vi "DrugControllerMain.vi"() -> ()   [LabVIEW 2019]
uses:
  DrugDosageTimeStampReference.ctl
panel:
  in  "TimeSimulator":dbl(slide) scale=0.0..24.0
  in  "Show Status":bool
  in  "Start":bool
  in  "Max Booster Allowed":u32 max=2
  in  "Planned Dosages":u32 max=10
  in  "Patient Name":string
  in  "Drug Id":string
  in  "Patient Id":string
  in  "Set Schedule":bool
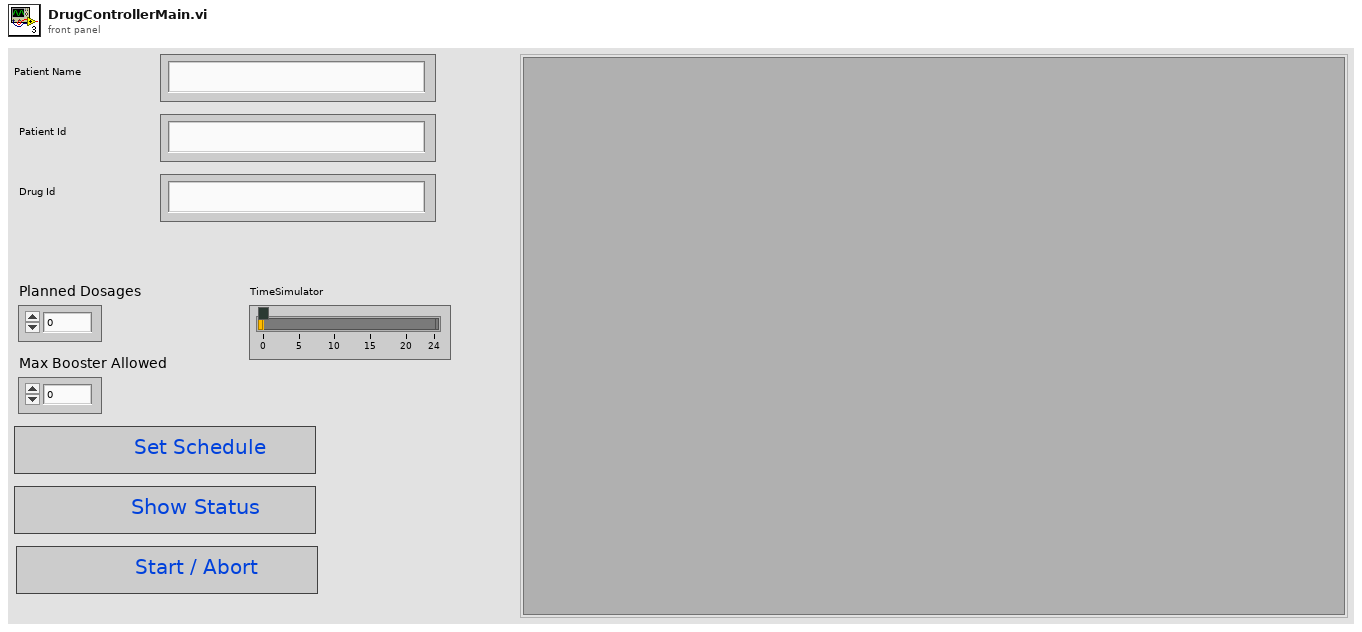
[diagram p1: front panel]
types:
  T1 = typedef "DrugDosageTimeStampReference.ctl" = cluster{"TimeStampControlReference":refnum<vi>, "DosageTime":timestamp}
  T2 = enum8{"Enabled", "Disabled", "Disabled and Grayed Out"}
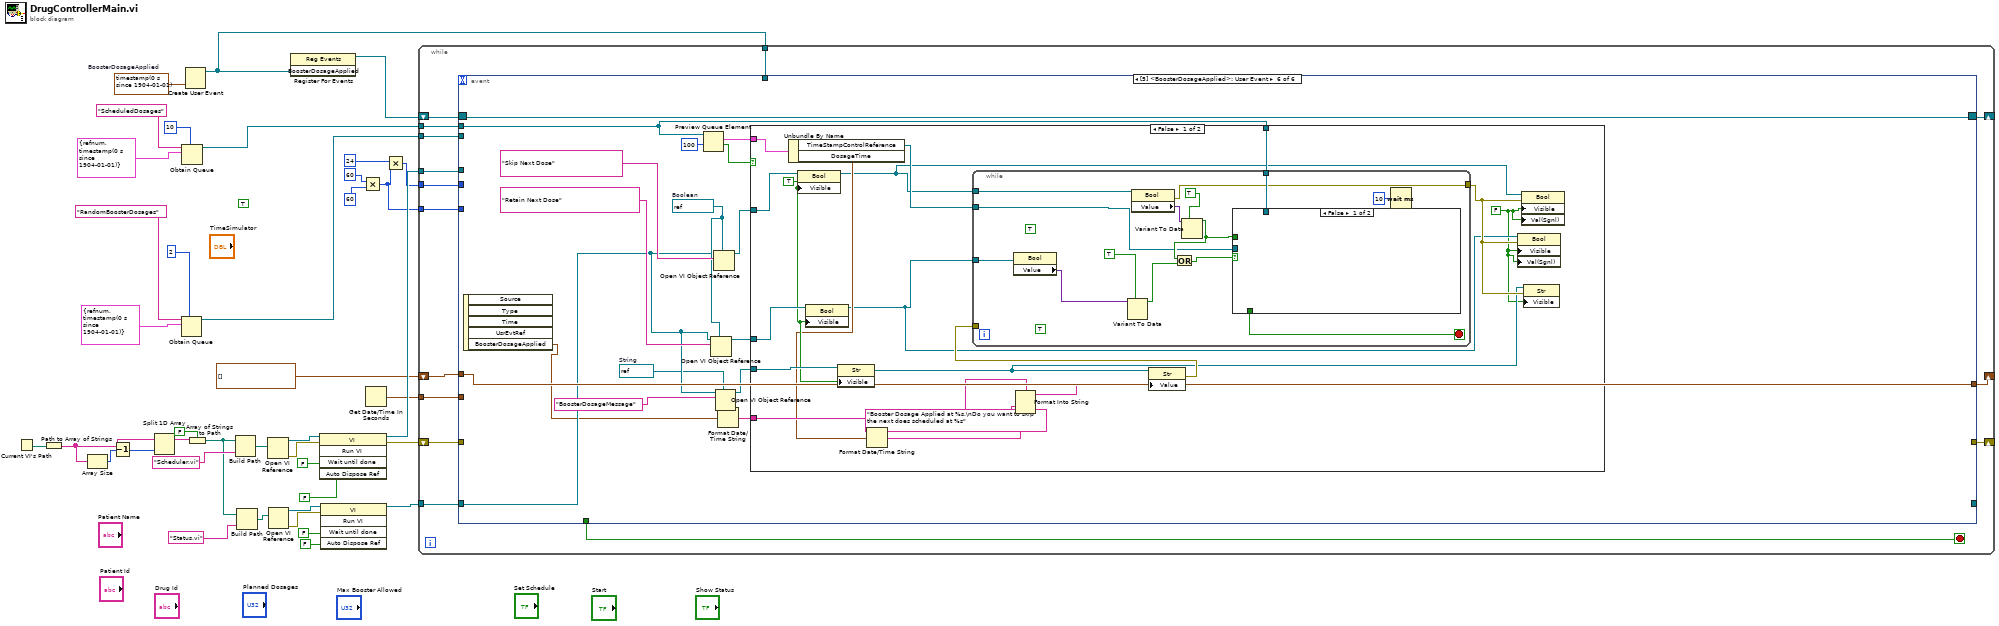
[diagram p0: block diagram]
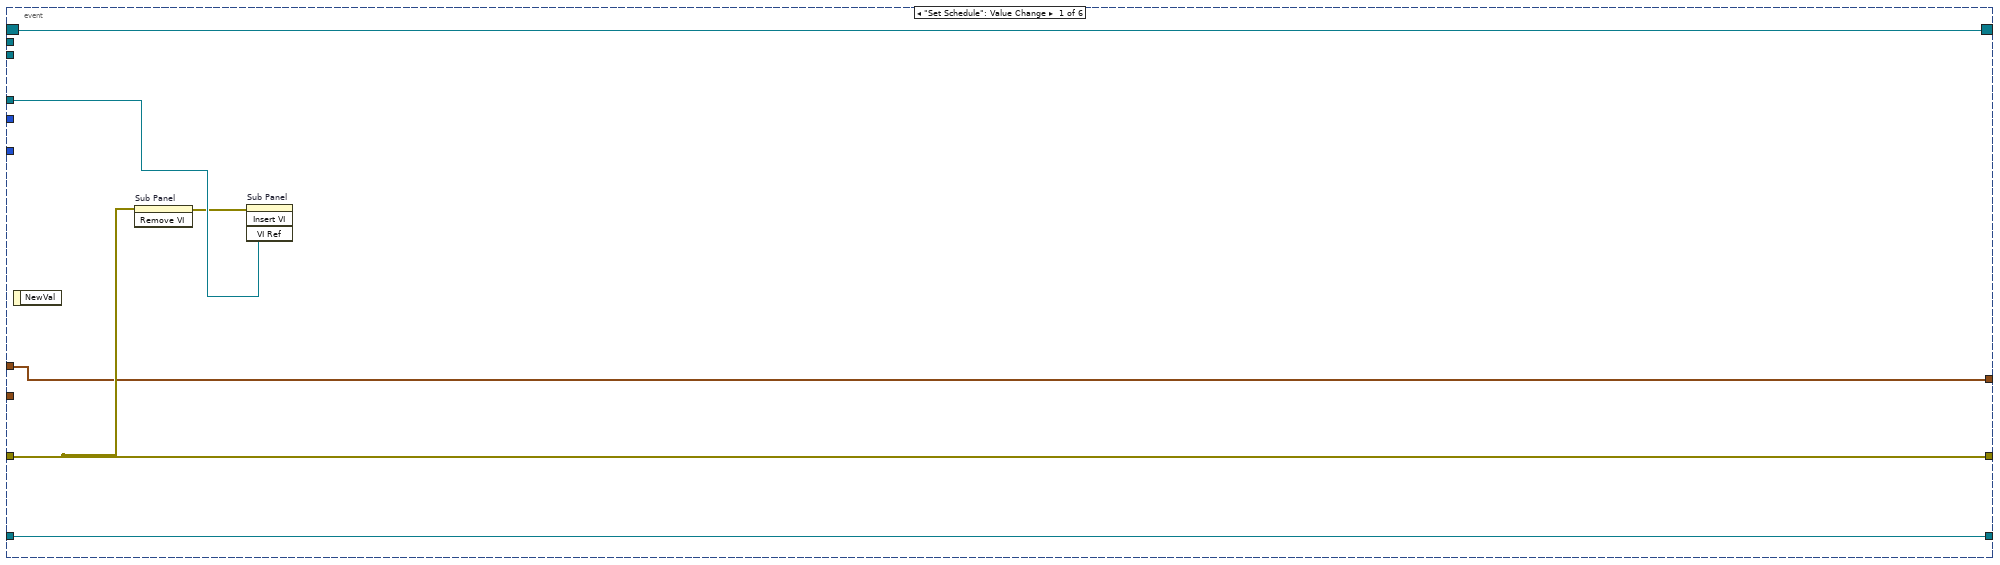
[diagram p2: hidden frame]
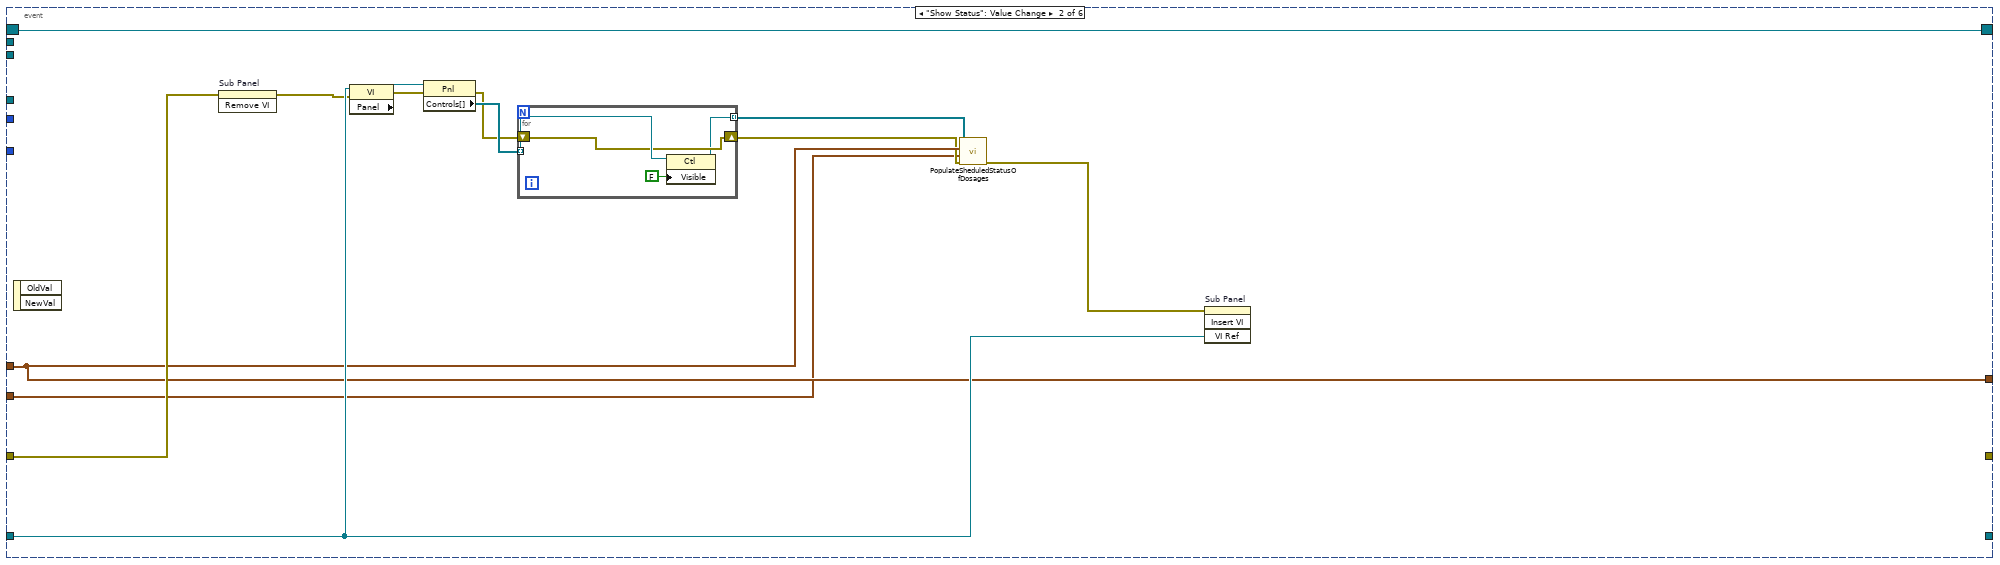
[diagram p3: hidden frame]
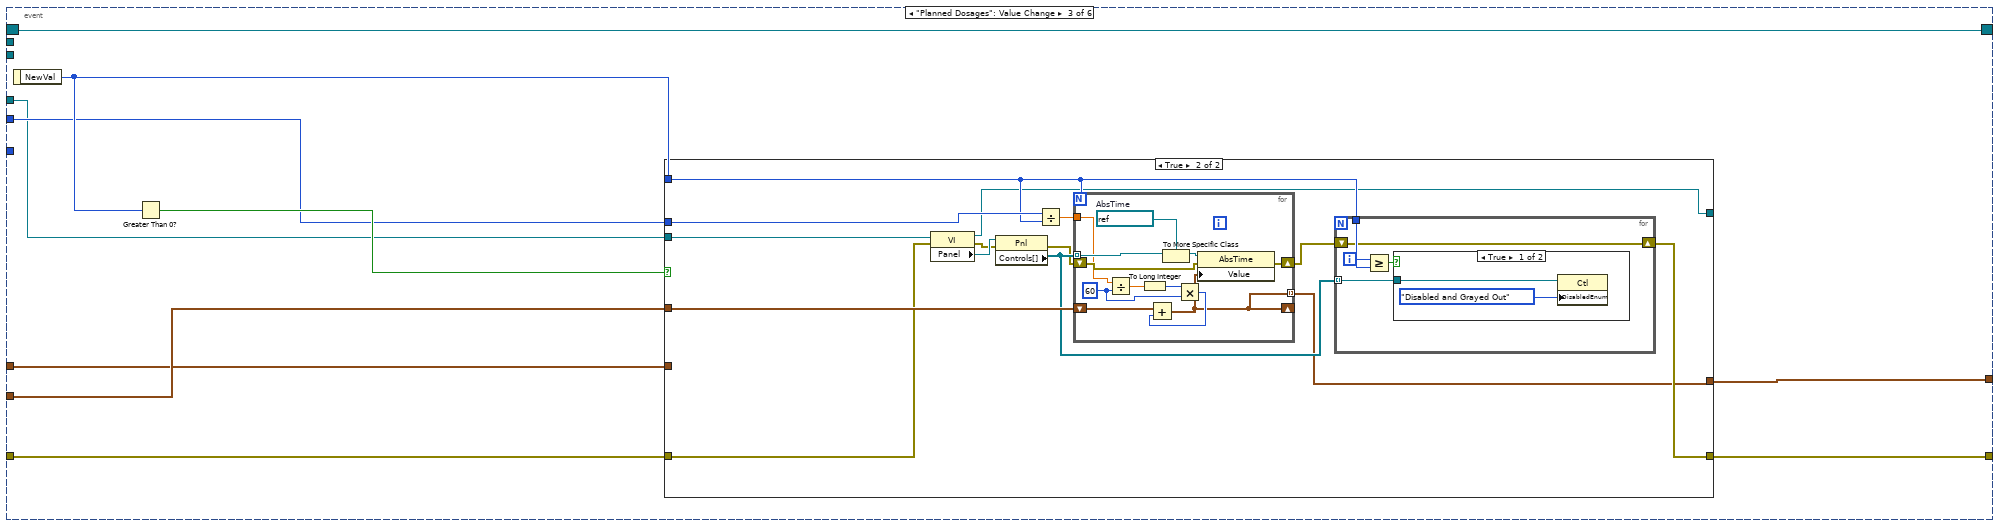
[diagram p4: hidden frame]
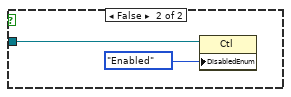
[diagram p6: hidden frame]
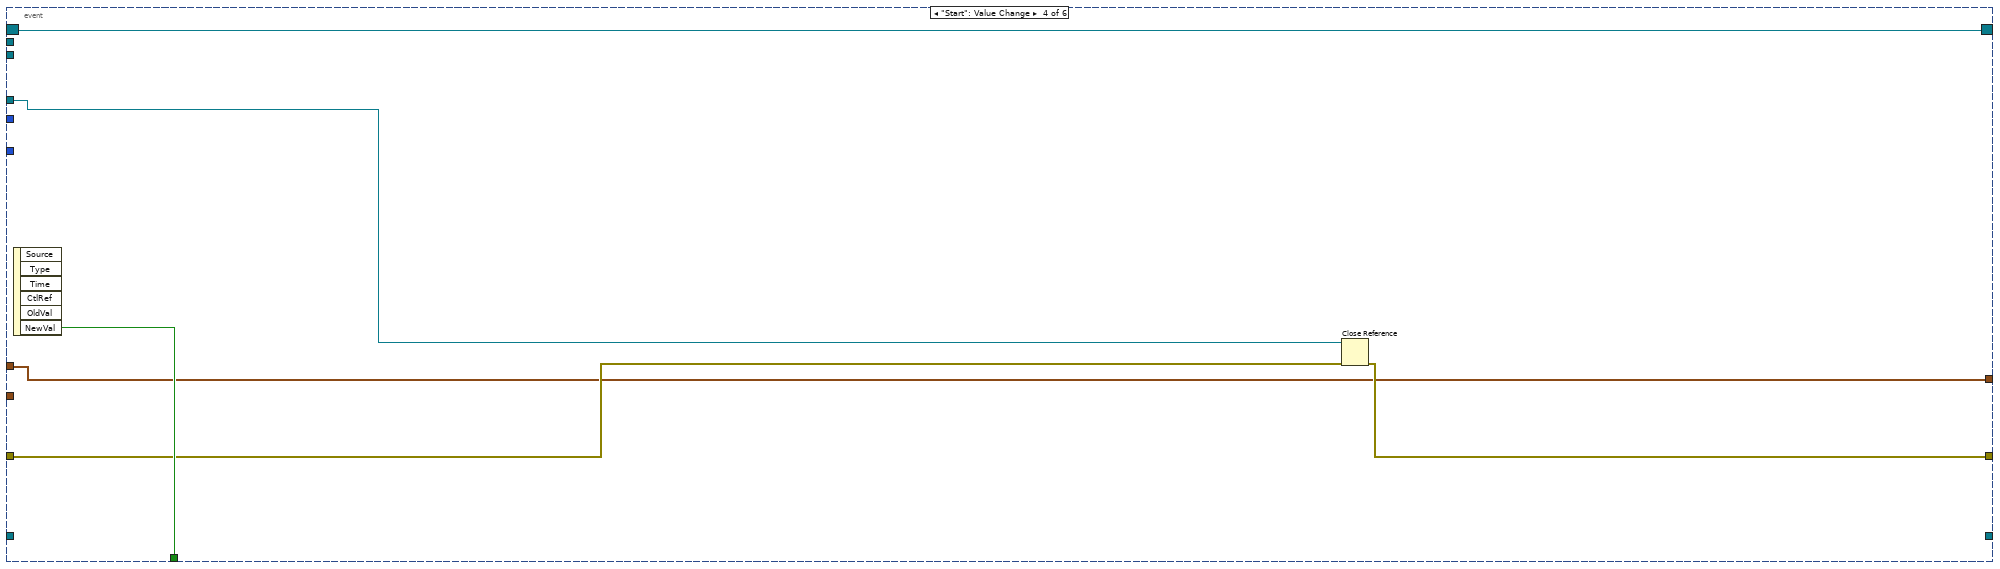
[diagram p7: hidden frame]
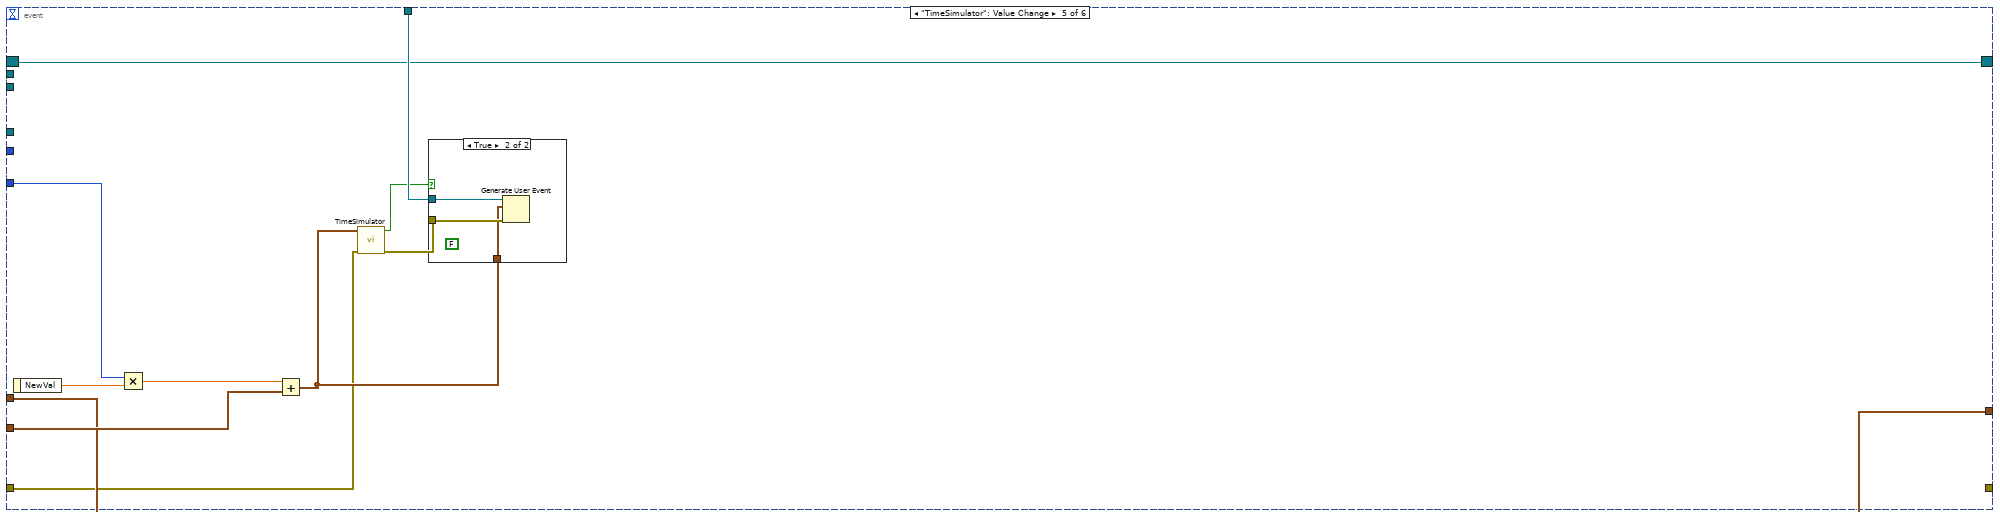
[diagram p8: hidden frame]
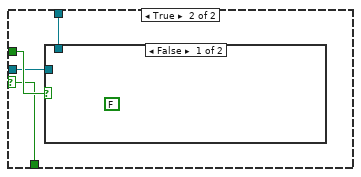
[diagram p10: hidden frame]
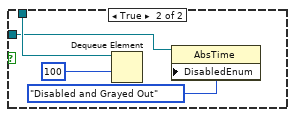
[diagram p11: hidden frame]
diagram:
  w10 = timestamp(0 s since 1904-01-01)  # BoosterDosageApplied
  (unwired) TRUE
  n1 = Current VI's Path() -> (path=w33:path)
  n2 = Path to Array of Strings(0:w33) -> (2:w35:string[])  [unwired: 1 out]
  n3 = Array Size(array=w35) -> (size(s)=w34:i32)
  n4 = Decrement(x=w34) -> (x-1=w37:i32)
  n5 = Split 1D Array(array=w35, index=w37) -> (first subarray=w38:string[])  [unwired: 1 out]
  n6 = Obtain Queue(max queue size (-1, unlimited)=2, name (unnamed)="RandomBoosterDosages", element data type=T1 {"TimeStampControlReference"=refnum, "DosageTime"=timestamp(0 s since 1904-01-01)}) -> (queue out=w1:refnum<queue>)  [unwired: 2 in, 2 out]
  n7 = Obtain Queue(max queue size (-1, unlimited)=10, name (unnamed)="ScheduledDosages", element data type=T1 {"TimeStampControlReference"=refnum, "DosageTime"=timestamp(0 s since 1904-01-01)}) -> (queue out=w6:refnum<queue>)  [unwired: 2 in, 2 out]
  n8 = Create User Event(user event datatype=w10) -> (user event=w9:refnum<user-event>)  [unwired: 1 in, 1 out]
  n9 = Array of Strings to Path(0:w38, 1:FALSE ("relative")) -> (2:w19:path)
  n10 = Build Path(base path=w19, name or relative path="Scheduler.vi") -> (appended path=w36:path)
  n11 = Build Path(base path=w19, name or relative path="Status.vi") -> (appended path=w20:path)
  n12 = Open VI Reference(vi path=w36) -> (vi reference=w27:refnum<vi>, error out=w28:errorcluster)  [unwired: 5 in]
  n13 = Open VI Reference(vi path=w20) -> (vi reference=w24:refnum<vi>, error out=w23:errorcluster)  [unwired: 5 in]
  n14 = register-events(w9) -> (reference out=w11:refnum<event-registration>)  [unwired: 2 in, 1 out]
  n15 = invoke class="VI" method="Run VI"(reference=w27, error in=w28, "Wait until done"=FALSE ("Wait Until Done"), "Auto Dispose Ref"=FALSE ("Auto Dispose Reference")) -> (reference out=w26:refnum<vi>, error out=w25:errorcluster)  [unwired: 1 in, 3 out]
  n16 = invoke class="VI" method="Run VI"(reference=w24, error in=w23, "Wait until done"=FALSE ("Wait Until Done"), "Auto Dispose Ref"=FALSE ("Auto Dispose Reference")) -> (reference out=w17:refnum<vi>)  [unwired: 1 in, 4 out]
  n17 = Multiply(x=60, y=60) -> (x*y=w14:i32)
  n18 = Get Date/Time In Seconds() -> (seconds since 1Jan1904=w12:timestamp)
  n19 = Multiply(x=24, y=w14) -> (x*y=w15:i32)
  n20 = while {
    tunnel: w15 -> [w54]
    shift-right: [w52] -> _
    shift-left: w25 -> [w51]
    tunnel: w17 -> [w50]
    tunnel: w26 -> [w53]
    tunnel: w14 -> [w49]
    tunnel: w12 -> [w48]
    shift-right: [w47] -> _
    shift-left: timestamp[] [] -> [w46]
    tunnel: w9 -> [w44]
    shift-right: [w43] -> _
    shift-left: w11 -> [w45]
    tunnel: w6 -> [w42]
    tunnel: w1 -> [w41]
    stop <- w55 stop-if-true
    n21 = event shown="[5] <BoosterDosageApplied>: User Event" {
      selector: w45 -> [w56 w62 w79 w127 w135 w162]
      dyn-events: [w56 w62 w79 w127 w135 w162] -> w43
      timeout: _ -> [_ _ _ _ _ _]
      tunnel: [_ _ _ w132 _ _] -> w55
      tunnel: w54 -> [_ _ w86 _ _ _]
      tunnel: w53 -> [w61 _ w85 w130 _ _]
      tunnel: [w60 _ w84 w131 _ _] -> w52
      tunnel: w51 -> [w60 w74 w83 w129 w133 _]
      tunnel: w50 -> [w57 w71 _ _ _ w152]
      tunnel: w49 -> [_ _ _ _ w143 _]
      tunnel: w48 -> [_ w63 w82 _ w141 _]
      tunnel: [w58 w69 w81 w128 w139 w163] -> w47
      tunnel: w46 -> [w58 w69 w80 w128 w139 w163]
      tunnel: [w57 _ _ _ _ _] -> _
      tunnel: w44 -> [_ _ _ _ w136 _]
      tunnel: w42 -> [_ _ _ _ _ w147]
      tunnel: w41 -> [_ _ _ _ _ _]
      event "Set Schedule": Value Change {
        n22 = event-data() -> ()  [unwired: 1 in, 1 out]
        n23 = invoke on="Sub Panel" class="SubPnl" method="Remove VI"(error in=w60) -> (error out=w59:errorcluster)  [unwired: 2 in, 2 out]
        n24 = invoke on="Sub Panel" class="SubPnl" method="Insert VI"(error in=w59, "VI Ref"=w61) -> ()  [unwired: 2 in, 4 out]
      }
      event "Show Status": Value Change {
        n25 = event-data() -> ()  [unwired: 1 in, 2 out]
        n26 = invoke on="Sub Panel" class="SubPnl" method="Remove VI"(error in=w74) -> (error out=w68:errorcluster)  [unwired: 2 in, 2 out]
        n27 = property class="VI"(reference=w71, error in=w68) -> (error out=w72:errorcluster, "Panel"=w73:refnum<vi>)  [unwired: 1 out]
        n28 = property class="Pnl"(reference=w73, error in=w72) -> (error out=w67:errorcluster, "Controls[]"=w70:refnum<vi>[])  [unwired: 1 out]
        n29 = for {
          tunnel: w70 -> [w78] mode=indexing
          tunnel: [w75] -> w64 mode=indexing
          shift-right: [w76] -> w66
          shift-left: w67 -> [w76]
          n30 = property class="Ctl"(reference=w78, "Visible"=FALSE) -> (reference out=w75:refnum<vi>)  [unwired: 1 in, 1 out]
        }
        n31 = call "PopulateSheduledStatusOfDosages.vi"("error in"=w66, "StartTimeOfDrugController"=w63, "Array"=w69, "Array 2"=w64) -> ("error out"=w65:errorcluster)  [unwired: 7 in]
        n32 = invoke on="Sub Panel" class="SubPnl" method="Insert VI"(error in=w65, "VI Ref"=w71) -> ()  [unwired: 2 in, 4 out]
      }
      event "Planned Dosages": Value Change {
        n33 = event-data() -> ("NewVal"=w88:u32)  [unwired: 1 in]
        n34 = Greater Than 0?(x=w88) -> (x > 0?=w87:bool)
        n35 = case shown="True" w87 {
          tunnel: w85 -> [w91 w99]
          tunnel: w88 -> [_ w100]
          tunnel: w86 -> [_ w105]
          tunnel: w82 -> [_ w104]
          tunnel: [w91 w97] -> _
          tunnel: [w90 w94] -> w84
          tunnel: w83 -> [w90 w93]
          tunnel: [w89 w92] -> w81
          tunnel: w80 -> [w89 _]
          frame False {
          }
          frame True {
            n36 = property class="VI"(reference=w99, error in=w93) -> (reference out=w97:refnum<vi>, error out=w96:errorcluster, "Panel"=w98:refnum<vi>)
            n37 = property class="Pnl"(reference=w98, error in=w96) -> (error out=w95:errorcluster, "Controls[]"=w102:refnum<vi>[])  [unwired: 1 out]
            n38 = Divide(x=w105, y=w100) -> (x/y=w103:dbl)
            n39 = for {
              N: w100 -> [_]
              tunnel: w102 -> [w125] mode=indexing
              tunnel: w103 -> [w120]
              shift-right: [w115] -> _
              shift-left: w104 -> [w123]
              shift-right: [w122] -> w101
              shift-left: w95 -> [w121]
              tunnel: [w115] -> w92 mode=indexing
              w117 = 60 ("y")
              w126 = refnum<vi> refnum  # AbsTime
              n40 = Divide(x=w120, y=w117) -> (x/y=w119:dbl)
              n41 = To Long Integer(number=w119) -> (32bit integer=w118:i32)
              n42 = To More Specific Class(target class=w126, reference=w125) -> (specific class reference=w124:refnum<vi>)  [unwired: 1 in, 1 out]
              n43 = Multiply(x=w118, y=w117) -> (x*y=w116:i32)
              n44 = Add(x=w123, y=w116) -> (x+y=w115:timestamp)
              n45 = property class="AbsTime"(reference=w124, error in=w121, "Value"=w115) -> (error out=w122:errorcluster)  [unwired: 1 out]
            }
            n46 = for {
              tunnel: w102 -> [w107] mode=indexing
              tunnel: w100 -> [w108]
              shift-right: [w106] -> w94
              shift-left: w101 -> [w106]
              i -> [w109]
              n47 = Greater Or Equal?(x=w109, y=w108) -> (x >= y?=w110:bool)
              n48 = case shown="True" w110 {
                tunnel: w107 -> [w112 w114]
                frame True {
                  n49 = property class="Ctl"(reference=w112, "DisabledEnum"=T2."Disabled and Grayed Out" ("Disabled")) -> ()  [unwired: 1 in, 2 out]
                }
                frame False {
                  n50 = property class="Ctl"(reference=w114, "DisabledEnum"=T2."Enabled" ("Disabled")) -> ()  [unwired: 1 in, 2 out]
                }
              }
            }
          }
        }
      }
      event "Start": Value Change {
        n51 = event-data() -> ("NewVal"=w132:bool)  [unwired: 1 in, 5 out]
        n52 = Close Reference(reference=w130, error in (no error)=w129) -> (error out=w131:errorcluster)
      }
      event "TimeSimulator": Value Change {
        n53 = event-data() -> ("NewVal"=w142:dbl)  [unwired: 1 in]
        n54 = Multiply(x=w143, y=w142) -> (x*y=w140:dbl)
        n55 = Add(x=w140, y=w141) -> (x+y=w137:timestamp)
        n56 = call "TimeSimulator.vi"("error in"=w133, "Time Stamp"=w137) -> ("error in 2"=w138:errorcluster, "BoosterDoseTriggerred"=w134:bool)  [unwired: 7 in, 1 out]
        n57 = case shown="True" w134 {
          tunnel: w138 -> [_ w146]
          tunnel: w137 -> [_ w145]
          tunnel: w136 -> [_ w144]
          frame False {
          }
          frame True {
            (unwired) FALSE
            n58 = Generate User Event(user event=w144, event data cluster=w145, error in=w146) -> ()  [unwired: 1 in, 2 out]
          }
        }
      }
      event User Event {
        w151 = refnum<vi> refnum  # String
        w156 = refnum<vi> refnum  # Boolean
        n59 = event-data() -> ("BoosterDosageApplied"=w149:timestamp)  [unwired: 1 in, 4 out]
        n60 = Preview Queue Element(queue=w147, timeout in ms (-1)=100) -> (element=w157:T1, timed out?=w159:bool)  [unwired: 1 in, 2 out]
        n61 = Open VI Object Reference(7:w156, 10:"Retain Next Dose" ("name/order"), 11:w152) -> (3:w154:refnum<vi>)  [unwired: 1 in, 1 out]
        n62 = Open VI Object Reference(7:w156, 10:"Skip Next Dose" ("name/order"), 11:w152) -> (3:w158:refnum<vi>)  [unwired: 1 in, 1 out]
        n63 = Open VI Object Reference(7:w151, 10:"BoosterDosageMessage" ("name/order"), 11:w152) -> (3:w150:refnum<vi>)  [unwired: 1 in, 1 out]
        n64 = Format Date/Time String(seconds (now)=w149) -> (date/time string=w148:string)  [unwired: 2 in]
        n65 = case shown="False" w159 {
          tunnel: w158 -> [w181 _]
          tunnel: w157 -> [w180 _]
          tunnel: w154 -> [w178 _]
          tunnel: w150 -> [w177 _]
          tunnel: w148 -> [w173 _]
          tunnel: w147 -> [w169 _]
          frame False {
            w164 = FALSE ("Visible")
            w176 = TRUE ("Visible")
            n66 = Unbundle By Name(w180) -> ("TimeStampControlReference"=w179:refnum<vi>, "DosageTime"=w172:timestamp)
            n67 = property class="Bool"(reference=w181, "Visible"=w176) -> (reference out=w168:refnum<vi>)  [unwired: 1 in, 1 out]
            n68 = property class="Bool"(reference=w178, "Visible"=w176) -> (reference out=w165:refnum<vi>)  [unwired: 1 in, 1 out]
            n69 = property class="Str"(reference=w177, "Visible"=w176) -> (reference out=w166:refnum<vi>)  [unwired: 1 in, 1 out]
            n70 = Format Date/Time String(seconds (now)=w172) -> (date/time string=w171:string)  [unwired: 2 in]
            n71 = Format Into String(format string="Booster Dosage Applied at %s.\nDo you want to skip the next does scheduled at %s" ("Value"), w173, w171) -> (resulting string=w174:string)  [unwired: 2 in, 1 out]
            n72 = property class="Str"(reference=w166, "Value"=w174) -> (error out=w170:errorcluster)  [unwired: 1 in, 1 out]
            n73 = while {
              tunnel: w168 -> [w195]
              tunnel: w179 -> [w182]
              tunnel: w165 -> [w193]
              tunnel: w170 -> [_]
              tunnel: w169 -> [w185]
              tunnel: [w183] -> w167
              stop <- w184 stop-if-true
              (unwired) TRUE
              (unwired) TRUE ("Blinking")
              n74 = property class="Bool"(reference=w193) -> ("Value"=w190:variant)  [unwired: 1 in, 2 out]
              n75 = Variant To Data(type=TRUE, Variant=w190) -> (data=w188:bool)  [unwired: 1 in, 1 out]
              n76 = property class="Bool"(reference=w195) -> (error out=w183:errorcluster, "Value"=w192:variant)  [unwired: 1 in, 1 out]
              n77 = Variant To Data(type=TRUE, Variant=w192) -> (data=w186:bool)  [unwired: 1 in, 1 out]
              n78 = Or(x=w186, y=w188) -> (x .or. y?=w187:bool)
              n79 = case shown="False" w187 {
                selector: w187 -> [_ w196]
                tunnel: w186 -> [_ w198]
                tunnel: w185 -> [_ w199]
                tunnel: w182 -> [_ w197]
                tunnel: [_ w196] -> w184
                frame False {
                }
                frame True {
                  n80 = case shown="False" w198 {
                    tunnel: w199 -> [_ w202]
                    tunnel: w197 -> [_ w201]
                    frame False {
                      (unwired) FALSE ("Blinking")
                    }
                    frame True {
                      n81 = Dequeue Element(queue=w202, timeout in ms (-1)=100) -> ()  [unwired: 1 in, 4 out]
                      n82 = property class="AbsTime"(reference=w201, "DisabledEnum"=T2."Disabled and Grayed Out" ("Disabled")) -> ()  [unwired: 1 in, 2 out]
                    }
                  }
                }
              }
              n83 = Wait (ms)(milliseconds to wait=u32 10) -> ()  [unwired: 1 out]
            }
            n84 = property class="Bool"(reference=w165, error in=w167, "Visible"=w164, "Val(Sgnl)"=w164) -> ()  [unwired: 2 out]
            n85 = property class="Bool"(reference=w168, error in=w167, "Visible"=w164, "Val(Sgnl)"=w164) -> ()  [unwired: 2 out]
            n86 = property class="Str"(reference=w166, error in=w167, "Visible"=w164) -> ()  [unwired: 2 out]
          }
          frame True {
          }
        }
      }
    }
  }
